vi "AD7747_Init.vi"(8 "error in":errorcluster) -> (0 "error out":errorcluster)   [LabVIEW 2012]
panel:
  # "Initialize AD7747 for Capacitance Measurement Mode"
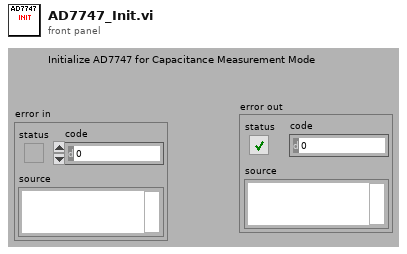
[diagram p1: front panel]
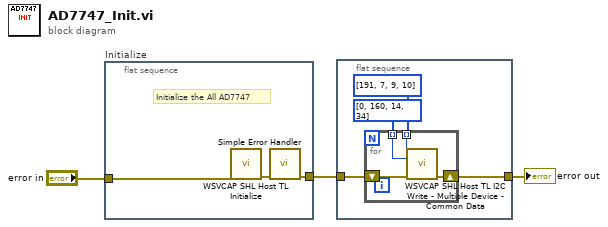
[diagram p0: block diagram]
diagram:
  n1 = flat-sequence "Initialize" {
    tunnel: "error in" -> [w4]
    tunnel: [w5] -> w2
    frame #0 {
      # "Initialize the All AD7747"
      n2 = call "WSVCAP SHL Host TL Initialize.vi"("error in"=w4) -> ("error out"=w6:errorcluster)  [unwired: 14 in]
      n3 = call <vilib>:"Simple Error Handler.vi"("error in (no error)"=w6) -> ("error out"=w5:errorcluster)  [unwired: 4 in, 4 out]
    }
  }
  n4 = flat-sequence {
    tunnel: w2 -> [w8]
    tunnel: [w7] -> w1
    frame #0 {
      n5 = for {
        tunnel: u8[] [191, 7, 9, 10] -> [w14] mode=indexing
        tunnel: u8[] [0, 160, 14, 34] -> [w13] mode=indexing
        shift-right: [w12] -> w7
        shift-left: w8 -> [w11]
        n6 = call "WSVCAP SHL Host TL I2C Write - Multiple Device - Common Data.vi"("Sub Address"=w14, "Data Out [U8]"=w13, "error in"=w11) -> ("error out"=w12:errorcluster)  [unwired: 12 in]
      }
    }
  }
  "error out" <- w1
